vi "organizeBufferToVolumeForDisplay.vi"(9 "xyz mode":bool, 10 "buffer":u32[](array[numeric]), 11 "volume info":T1) -> (1 "fb only (image if no ff/fb)":u32[][][](array[numeric]), 2 "ff only (0 if no ff/fb)":u32[][][](array[numeric]), 3 "image":u32[][][](array[numeric]))   [LabVIEW 2010]
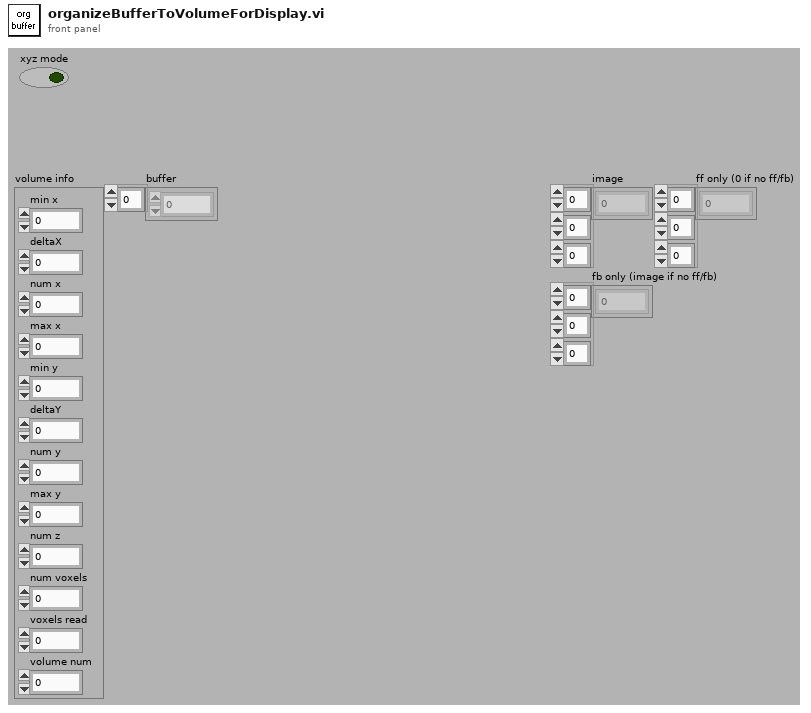
[diagram p1: front panel]
types:
  T1 = cluster{"min x":i16, "deltaX":dbl, "num x":u32, "max x":i16, "min y":i16, "deltaY":dbl, "num y":u32, "max y":i16, "num z":u32, "num voxels":u32, "voxels read":u32, "volume num":u32}
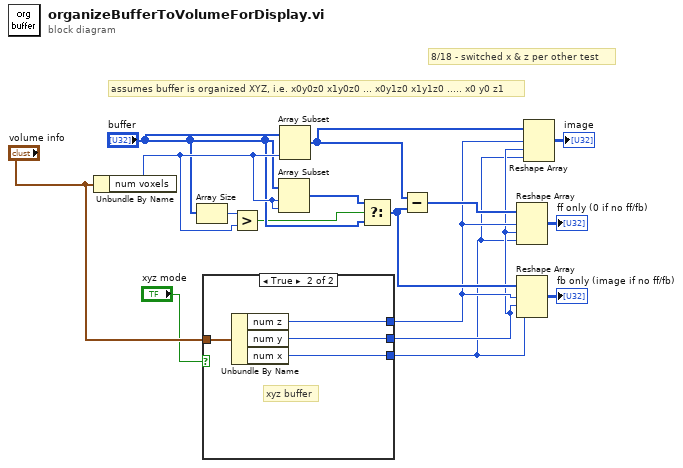
[diagram p0: block diagram]
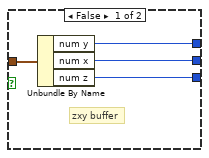
[diagram p2: hidden frame]
diagram:
  # "assumes buffer is organized XYZ, i.e. x0y0z0 x1y0z0 ... x0y1z0 x1y1z0 ..... x0 y0 z1"
  # "8/18 - switched x & z per other test"
  n1 = Unbundle By Name("volume info") -> ("num voxels"=w15:u32)
  n2 = Array Size(array="buffer") -> (size(s)=w16:i32)
  n3 = case shown="True" "xyz mode" {
    tunnel: "volume info" -> [w20 w24]
    tunnel: [w19 w23] -> w3
    tunnel: [w18 w22] -> w2
    tunnel: [w17 w21] -> w1
    frame False {
      # "zxy buffer"
      n4 = Unbundle By Name(w20) -> ("num y"=w19:u32, "num x"=w18:u32, "num z"=w17:u32)
    }
    frame True {
      # "xyz buffer"
      n5 = Unbundle By Name(w24) -> ("num z"=w23:u32, "num y"=w22:u32, "num x"=w21:u32)
    }
  }
  n6 = Greater?(x=w16, y=w15) -> (0:w12:bool)
  n7 = Array Subset(array="buffer", index=w15, length=w15) -> (w14:u32[])
  n8 = Array Subset(array="buffer", length=w15) -> (w11:u32[])  [unwired: 1 in]
  n9 = Select(t=w14, s=w12, f="buffer") -> (s? t:f=w10:u32[])
  n10 = Subtract(x=w11, y=w10) -> (x-y=w5:u32[])
  n11 = Reshape Array(w5, w3, w2, w1) -> (→"ff only (0 if no ff/fb)":u32[][][])
  n12 = Reshape Array(w10, w3, w2, w1) -> (→"fb only (image if no ff/fb)":u32[][][])
  n13 = Reshape Array(w11, w3, w2, w1) -> (→"image":u32[][][])
